vi "Pointer producer consumer From Hexa Convertor.vi"(11 "string":string) -> (0 "Voltage on ADC3":dbl, 1 "Voltage on ADC2":dbl, 2 "Voltage on ADC1":dbl, 3 "Voltage on ADC0":dbl)   [LabVIEW 2014]
doc: "prevadza prijaty retazec znakov na napatie zosnimane ADC prevodnikom"
panel:
  in  "V / mV":bool
  out "ADC3":u32
  out "ADC2":u32
  out "ADC1":u32
  out "ADC0":u32
  out "dataH3":u32
  out "dataL3":u32
  out "dataH2":u32
  out "dataL2":u32
  out "Array (Hexa)":string[](array[string])
  out "dataH1":u32
  out "dataL1":u32
  out "dataH0":u32
  out "dataL0":u32
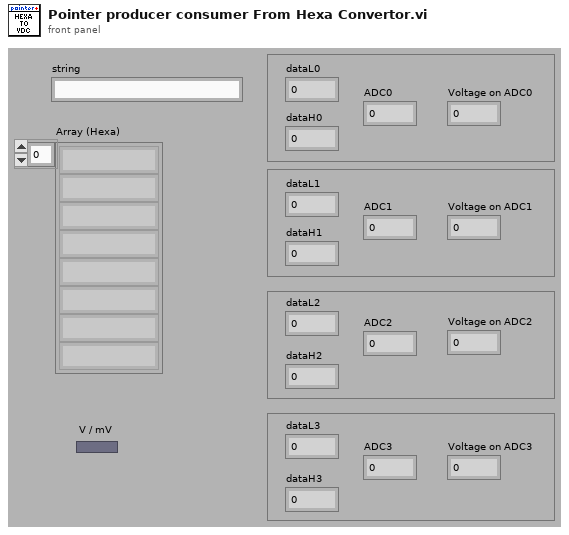
[diagram p1: front panel]
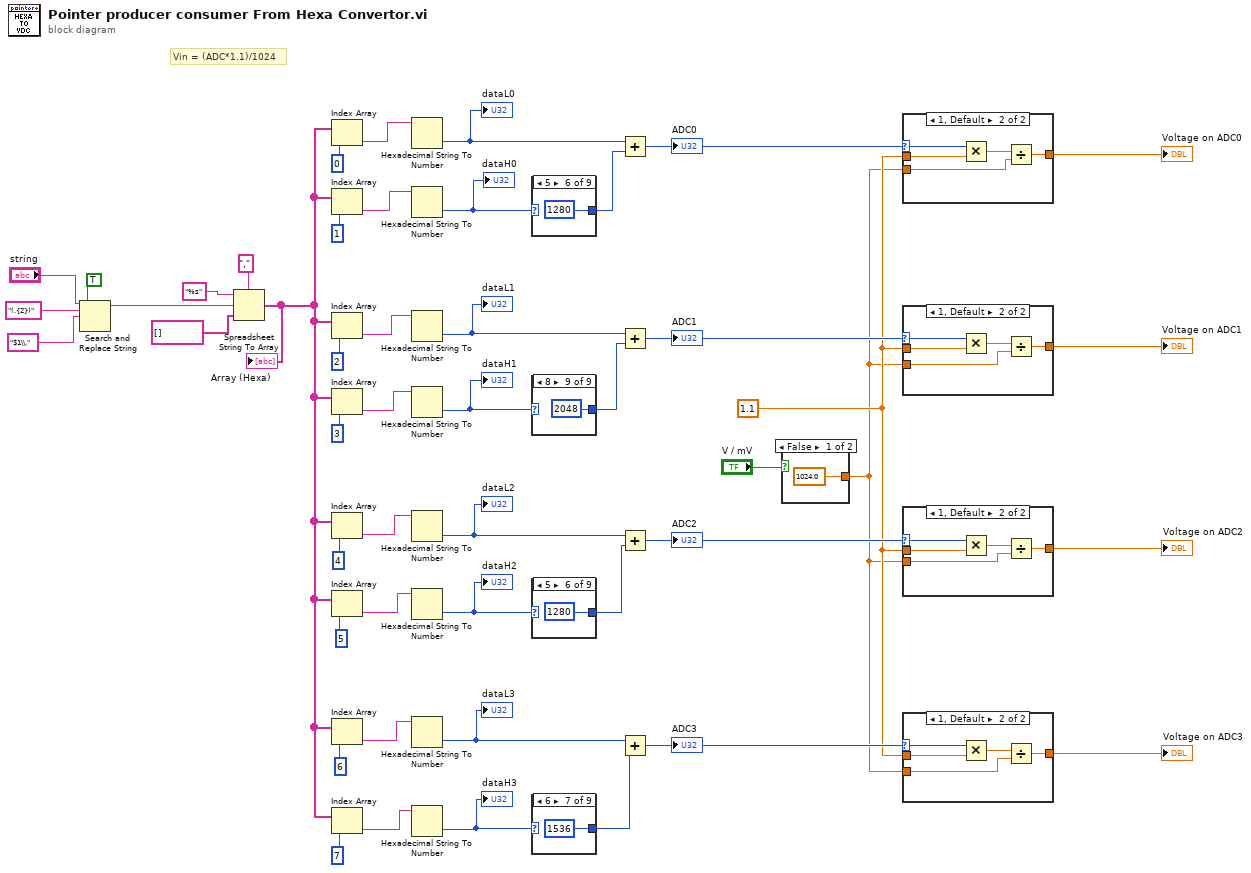
[diagram p0: block diagram]
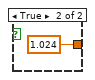
[diagram p2: hidden frame]
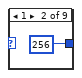
[diagram p4: hidden frame]
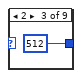
[diagram p5: hidden frame]
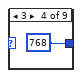
[diagram p6: hidden frame]
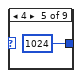
[diagram p7: hidden frame]
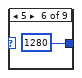
[diagram p8: hidden frame]
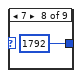
[diagram p9: hidden frame]
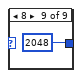
[diagram p10: hidden frame]
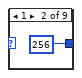
[diagram p13: hidden frame]
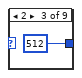
[diagram p14: hidden frame]
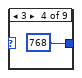
[diagram p15: hidden frame]
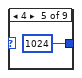
[diagram p16: hidden frame]
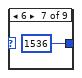
[diagram p17: hidden frame]
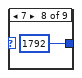
[diagram p18: hidden frame]
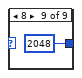
[diagram p19: hidden frame]
diagram:
  w6 = 1.1 ("y")
  # "Vin = (ADC*1.1)/1024"
  n1 = Search and Replace String(replace all?=TRUE, input string="string", search string="(.{2})", replace string="$1\\,") -> (result string=w42:string)  [unwired: 4 in, 3 out]
  n2 = Spreadsheet String To Array(delimiter (Tab)=",", format string="%s", spreadsheet string=w42, array type (2D Dbl)=string[] [] ("Array")) -> (array=w7:string[])
  "Array (Hexa)" <- w7
  n3 = Index Array(array=w7, index=0) -> (element=w38:string)
  n4 = Index Array(array=w7, index=1) -> (element=w37:string)
  n5 = Index Array(array=w7, index=2) -> (element=w34:string)
  n6 = Index Array(array=w7, index=3) -> (element=w33:string)
  n7 = Index Array(array=w7, index=4) -> (element=w31:string)
  n8 = Index Array(array=w7, index=5) -> (element=w29:string)
  n9 = Index Array(array=w7, index=6) -> (element=w27:string)
  n10 = Index Array(array=w7, index=7) -> (element=w25:string)
  n11 = Hexadecimal String To Number(string=w38) -> (number=w24:u32)  [unwired: 2 in, 1 out]
  "dataL0" <- w24
  n12 = Hexadecimal String To Number(string=w37) -> (number=w23:u32)  [unwired: 2 in, 1 out]
  "dataH0" <- w23
  n13 = Hexadecimal String To Number(string=w34) -> (number=w20:u32)  [unwired: 2 in, 1 out]
  "dataL1" <- w20
  n14 = Hexadecimal String To Number(string=w33) -> (number=w19:u32)  [unwired: 2 in, 1 out]
  "dataH1" <- w19
  n15 = Hexadecimal String To Number(string=w31) -> (number=w15:u32)  [unwired: 2 in, 1 out]
  "dataL2" <- w15
  n16 = Hexadecimal String To Number(string=w29) -> (number=w13:u32)  [unwired: 2 in, 1 out]
  "dataH2" <- w13
  n17 = Hexadecimal String To Number(string=w27) -> (number=w16:u32)  [unwired: 2 in, 1 out]
  "dataL3" <- w16
  n18 = Hexadecimal String To Number(string=w25) -> (number=w14:u32)  [unwired: 2 in, 1 out]
  "dataH3" <- w14
  n19 = case shown="5" w23 {
    selector: w23 -> [w49 _ _ _ _ _ _ _ _]
    tunnel: [w49 u32 256 u32 512 u32 768 u32 1024 u32 1280 u32 1536 u32 1792 u32 2048] -> w22
    frame 0, Default {
    }
    frame 1 {
    }
    frame 2 {
    }
    frame 3 {
    }
    frame 4 {
    }
    frame 5 {
    }
    frame 6 {
    }
    frame 7 {
    }
    frame 8 {
    }
  }
  n20 = case shown="8" w19 {
    selector: w19 -> [w58 _ _ _ _ _ _ _ _]
    tunnel: [w58 u32 256 u32 512 u32 768 u32 1024 u32 1280 u32 1536 u32 1792 u32 2048] -> w21
    frame 0, Default {
    }
    frame 1 {
    }
    frame 2 {
    }
    frame 3 {
    }
    frame 4 {
    }
    frame 5 {
    }
    frame 6 {
    }
    frame 7 {
    }
    frame 8 {
    }
  }
  n21 = case shown="5" w13 {
    selector: w13 -> [w67 _ _ _ _ _ _ _ _]
    tunnel: [w67 u32 256 u32 512 u32 768 u32 1024 u32 1280 u32 1536 u32 1792 u32 2048] -> w18
    frame 0, Default {
    }
    frame 1 {
    }
    frame 2 {
    }
    frame 3 {
    }
    frame 4 {
    }
    frame 5 {
    }
    frame 6 {
    }
    frame 7 {
    }
    frame 8 {
    }
  }
  n22 = case shown="6" w14 {
    selector: w14 -> [w76 _ _ _ _ _ _ _ _]
    tunnel: [w76 u32 256 u32 512 u32 768 u32 1024 u32 1280 u32 1536 u32 1792 u32 2048] -> w17
    frame 0, Default {
    }
    frame 1 {
    }
    frame 2 {
    }
    frame 3 {
    }
    frame 4 {
    }
    frame 5 {
    }
    frame 6 {
    }
    frame 7 {
    }
    frame 8 {
    }
  }
  n23 = Add(x=w24, y=w22) -> (x+y=w11:u32)
  "ADC0" <- w11
  n24 = Add(x=w20, y=w21) -> (x+y=w10:u32)
  "ADC1" <- w10
  n25 = Add(x=w15, y=w18) -> (x+y=w9:u32)
  "ADC2" <- w9
  n26 = Add(x=w16, y=w17) -> (x+y=w8:u32)
  "ADC3" <- w8
  n27 = case shown="False" "V / mV" {
    tunnel: [1024.0 ("y") 1.024 ("y")] -> w5
    frame False {
    }
    frame True {
    }
  }
  n28 = case shown="1, Default" w11 {
    selector: w11 -> [w87 w90]
    tunnel: [w87 w91] -> w4
    tunnel: w6 -> [_ w89]
    tunnel: w5 -> [_ w88]
    frame 0 {
    }
    frame 1, Default {
      n29 = Multiply(x=w90, y=w89) -> (x*y=w92:dbl)
      n30 = Divide(x=w92, y=w88) -> (x/y=w91:dbl)
    }
  }
  "Voltage on ADC0" <- w4
  n31 = case shown="1, Default" w10 {
    selector: w10 -> [w93 w96]
    tunnel: [w93 w97] -> w3
    tunnel: w6 -> [_ w95]
    tunnel: w5 -> [_ w94]
    frame 0 {
    }
    frame 1, Default {
      n32 = Multiply(x=w96, y=w95) -> (x*y=w98:dbl)
      n33 = Divide(x=w98, y=w94) -> (x/y=w97:dbl)
    }
  }
  "Voltage on ADC1" <- w3
  n34 = case shown="1, Default" w9 {
    selector: w9 -> [w99 w102]
    tunnel: [w99 w103] -> w2
    tunnel: w6 -> [_ w101]
    tunnel: w5 -> [_ w100]
    frame 0 {
    }
    frame 1, Default {
      n35 = Multiply(x=w102, y=w101) -> (x*y=w104:dbl)
      n36 = Divide(x=w104, y=w100) -> (x/y=w103:dbl)
    }
  }
  "Voltage on ADC2" <- w2
  n37 = case shown="1, Default" w8 {
    selector: w8 -> [w105 w108]
    tunnel: [w105 w109] -> w1
    tunnel: w6 -> [_ w107]
    tunnel: w5 -> [_ w106]
    frame 0 {
    }
    frame 1, Default {
      n38 = Multiply(x=w108, y=w107) -> (x*y=w110:dbl)
      n39 = Divide(x=w110, y=w106) -> (x/y=w109:dbl)
    }
  }
  "Voltage on ADC3" <- w1
